vi "DAQ_DO.vi"(6 "Slot":T1, 8 "error in":errorcluster, 10 "State":bool, 11 "DOCH":T2=enum."PowerON_+B") -> (0 "error out":errorcluster)   [LabVIEW 2013]
uses:
  SystemCode/SysControl/Slot.ctl
  <vilib>/DAQmx/write.llb/DAQmx Write (Digital Bool 1Line 1Point).vi
  <vilib>/DAQmx/read.llb/DAQmx Read (Digital Bool 1Line 1Point).vi
  SourceCode/GlobalValue.vi
  <vilib>/DAQmx/create/channels.llb/DAQmx Create Channel (DO-Digital Output).vi
  <vilib>/DAQmx/miscellaneous.llb/DAQmx Fill In Error Info.vi
panel:
  out "DO status":bool
  out "CH":string
  out "Line/port":tag="PCI-6229/port0/line0:1"
  in  "Enum":enum16{"Set", "Get", "Initialize"}(ring)
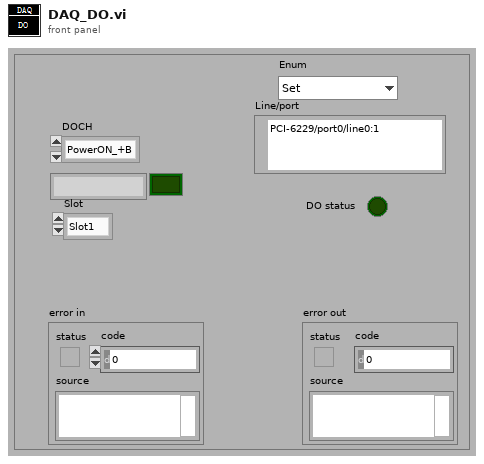
[diagram p1: front panel]
types:
  T1 = typedef "Slot.ctl" = enum16{"Slot1", "Slot2", "Slot3", "Slot4"}
  T2 = typedef "DO信号名称.ctl" = enum16{"ACC", "ILL", "BACK", "BRAKE", "PowerON_Vps", "PowerON_+B", "SW", "SW1", "SW2", "LineOut1", "LineOut2", "LineOut3", "LineOut4", "LineOut5", "LineOut6", "SPK", "SPK2", "IPOD_DET", "RING"}
  T3 = typedef "DAQConfig.ctl" = cluster{"DIO":string[][], "AO":string[][], "AI":string[][]}
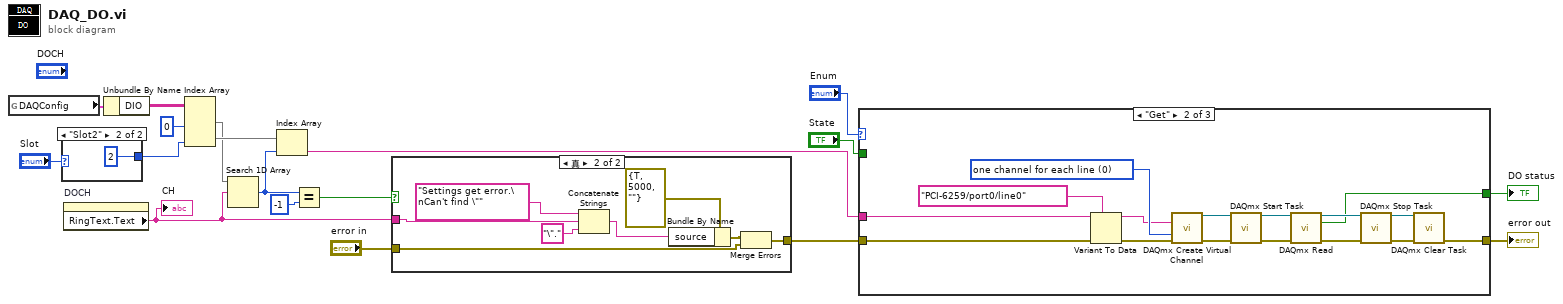
[diagram p0: block diagram]
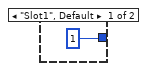
[diagram p2: hidden frame]
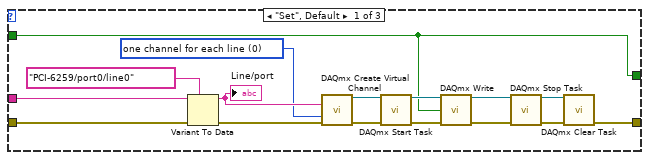
[diagram p4: hidden frame]
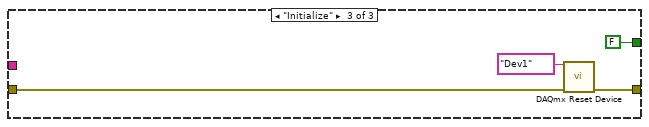
[diagram p5: hidden frame]
diagram:
  n1 = global read "GlobalValue.vi" "DAQConfig"() -> (w1:T3)
  n2 = case shown="\"Slot2\"" "Slot" {
    tunnel: [1 ("索引 (行)") 2 ("索引 (行)")] -> w2
    frame "Slot1", Default {
    }
    frame "Slot2" {
    }
  }
  n3 = property on="DOCH" class="Enum (严格)"() -> ("RingText.Text"=w4:string)  [unwired: 2 in, 2 out]
  "CH" <- w4
  n4 = Unbundle By Name(w1) -> ("DIO"=w16:string[][])
  n5 = Index Array(array=w16, index (col) #1=0 ("索引 (行)"), index (col) #2=w2) -> (element #1=w6:string[], element #2=w14:string[])  [unwired: 2 in]
  n6 = Search 1D Array(1D array=w6, element=w4) -> (index of element=w11:i32)  [unwired: 1 in]
  n7 = Index Array(array=w14, index=w11) -> (element=w17:string)
  n8 = Equal?(x=w11, y=-1) -> (x = y?=w9:bool)
  n9 = case shown="真" w9 {
    tunnel: w4 -> [_ w25]
    tunnel: "error in" -> [w21 w24]
    tunnel: [w21 w23] -> w5
    frame False {
    }
    frame True {
      n10 = Concatenate Strings("Settings get error.\nCan't find \"" ("message"), w25, "\"." ("string")) -> (w28:string)
      n11 = Bundle By Name(cluster=errorcluster {"status"=TRUE, "code"=5000, "source"=""} ("error in 1 (no error)"), "source"=w28) -> (w27:errorcluster)
      n12 = Merge Errors(w27, w24) -> (w23:errorcluster)
    }
  }
  n13 = case shown="\"Get\"" "Enum" {
    tunnel: w5 -> [w31 w46 w65]
    tunnel: [w39 w55 w64] -> w13
    tunnel: [w30 w48 FALSE ("data")] -> w7
    tunnel: w17 -> [w32 w47 _]
    tunnel: "State" -> [w30 _ _]
    frame "Set", Default {
      w34 = 0 items=["one channel for each line", "one channel for all lines"] ("line grouping")
      n14 = Variant To Data(error in=w31, type=tag "PCI-6259/port0/line0" ("lines"), Variant=w32) -> (data=w37:tag, error out=w33:errorcluster)
      "Line/port" <- w37
      n15 = call-poly <vilib>:"DAQmx Create Virtual Channel.vi"("lines"=w37, "line grouping"=w34, "error in"=w33) -> ("task out"=w45:refnum<k21>, "error out"=w44:errorcluster)  [unwired: 11 in]
      n16 = call <vilib>:"DAQmx Start Task.vi"("task/channels in"=w45, "error in"=w44) -> ("task out"=w43:refnum<k21>, "error out"=w42:errorcluster)  [unwired: 12 in]
      n17 = call-poly <vilib>:"DAQmx Write.vi"("task/channels in"=w43, "data"=w30, "error in"=w42) -> ("task out"=w36:refnum<k21>, "error out"=w35:errorcluster)  [unwired: 10 in, 1 out]
      n18 = call <vilib>:"DAQmx Stop Task.vi"("task/channels in"=w36, "error in"=w35) -> ("task out"=w41:refnum<k21>, "error out"=w40:errorcluster)  [unwired: 12 in]
      n19 = call <vilib>:"DAQmx Clear Task.vi"("task in"=w41, "error in"=w40) -> ("error out"=w39:errorcluster)  [unwired: 13 in]
    }
    frame "Get" {
      w54 = 0 items=["one channel for each line", "one channel for all lines"] ("line grouping")
      n20 = Variant To Data(error in=w46, type=tag "PCI-6259/port0/line0" ("lines"), Variant=w47) -> (data=w52:tag, error out=w51:errorcluster)
      n21 = call-poly <vilib>:"DAQmx Create Virtual Channel.vi"("lines"=w52, "line grouping"=w54, "error in"=w51) -> ("task out"=w61:refnum<k21>, "error out"=w60:errorcluster)  [unwired: 11 in]
      n22 = call <vilib>:"DAQmx Start Task.vi"("task/channels in"=w61, "error in"=w60) -> ("task out"=w59:refnum<k21>, "error out"=w58:errorcluster)  [unwired: 12 in]
      n23 = call-poly <vilib>:"DAQmx Read.vi"("task/channels in"=w59, "error in"=w58) -> ("task out"=w50:refnum<k21>, "data"=w48:bool, "error out"=w49:errorcluster)  [unwired: 11 in]
      n24 = call <vilib>:"DAQmx Stop Task.vi"("task/channels in"=w50, "error in"=w49) -> ("task out"=w57:refnum<k21>, "error out"=w56:errorcluster)  [unwired: 12 in]
      n25 = call <vilib>:"DAQmx Clear Task.vi"("task in"=w57, "error in"=w56) -> ("error out"=w55:errorcluster)  [unwired: 13 in]
    }
    frame "Initialize" {
      n26 = call <vilib>:"DAQmx Reset Device.vi"("device in"=tag "Dev1", "error in"=w65) -> ("error out"=w64:errorcluster)  [unwired: 13 in]
    }
  }
  "error out" <- w13
  "DO status" <- w7
